vi "Remove SRs.vi"(8 "error in (no error)":errorcluster, 9 "Array":i32[](array[numeric]), 11 "Data Loop Data in":T1) -> (0 "error out":errorcluster, 3 "Data Loop Data out":T1)   [LabVIEW 2018]
uses:
  Type Defs/Screenpop Loop Data.ctl
  Support/Message Queue/Message Cluster.ctl
  Type Defs/FGV States.ctl
  Support/Message Queue/Message Queue.lvlib
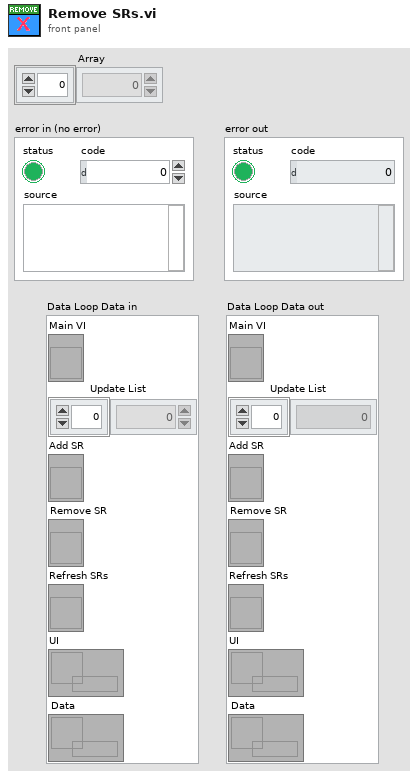
[diagram p1: front panel]
types:
  T1 = typedef "Screenpop Loop Data.ctl" = cluster{"Main VI":refnum<vi>, "Update List":i32[], "Add SR":refnum<vi>, "Remove SR":refnum<vi>, "Refresh SRs":refnum<vi>, "UI":refnum<queue>, "Data":refnum<queue>}
  T2 = typedef "FGV States.ctl" = enum16{"Initialize", "Merge", "Write", "Remove", "Read", "Clear"}
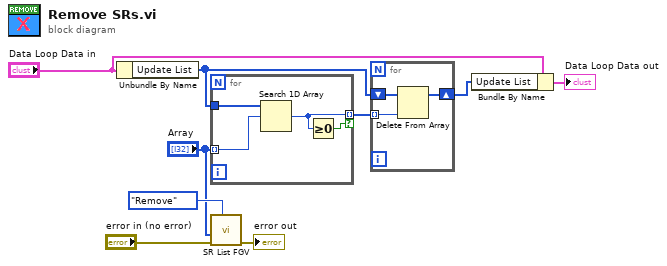
[diagram p0: block diagram]
diagram:
  n1 = Unbundle By Name("Data Loop Data in") -> ("Update List"=w3:i32[])
  n2 = for {
    tunnel: "Array" -> [w10] mode=indexing
    tunnel: w3 -> [w13]
    tunnel: [w12] -> w2 mode=indexing if=w11
    n3 = Search 1D Array(1D array=w13, element=w10) -> (index of element=w12:i32)  [unwired: 1 in]
    n4 = Greater Or Equal To 0?(x=w12) -> (x >= 0?=w11:bool)
  }
  n5 = call "SR List FGV.vi"("Operation"=FGV_States."Remove", "Error In"="error in (no error)", "Input"="Array") -> ("Error Out"=→"error out":errorcluster)  [unwired: 7 in, 1 out]
  n6 = for {
    tunnel: w2 -> [w15] mode=indexing
    shift-right: [w14] -> w4
    shift-left: w3 -> [w16]
    n7 = Delete From Array(array=w16, index=w15) -> (array with subset deleted=w14:i32[])  [unwired: 1 in, 1 out]
  }
  n8 = Bundle By Name(cluster="Data Loop Data in", "Update List"=w4) -> (→"Data Loop Data out":T1)
